vi "closeVISA.vi"() -> ()   [LabVIEW 2013]
panel:
  in  "test \nVISA Handle out 2":refnum<visa-resource-name>
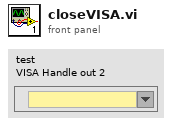
[diagram p1: front panel]
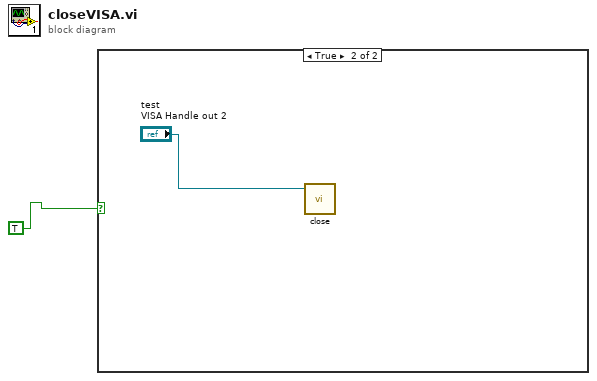
[diagram p0: block diagram]
diagram:
  n1 = case shown="True" TRUE {
    frame False {
    }
    frame True {
      n2 = call "close.vi"("VISA Handle in"="test \nVISA Handle out 2") -> ()  [unwired: 4 in, 1 out]
    }
  }
